vi "signal_analyze.vi"() -> ()   [LabVIEW 2021]
uses:
  <vilib>/express/express analysis/Spectral/Block/exnSpectralBlock spectral measurements power poly.vi
  <vilib>/express/express analysis/Spectral/Block/exnSpectralBlock spectral measurements power DDT.vi
  <vilib>/express/express analysis/Spectral/XNode/ExpressSpectralMeasurementsBlockNode.xnode
panel:
  in  "Stop":bool
  out "Waveform Graph":dynamicdata(graph)
  in  "Sine Frequency":dbl(knob) scale=0.0..500.0
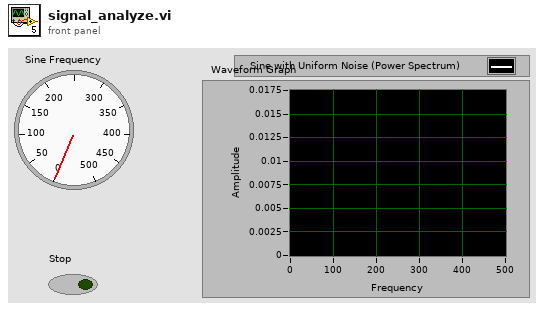
[diagram p1: front panel]
types:
  T1 = cluster{"averaging mode":u16, "weighting mode":u16, "number of averages":u32}
  T2 = cluster{"dB On (F)":bool, "unwrap phase (F)":bool, "convert to degree (F)":bool}
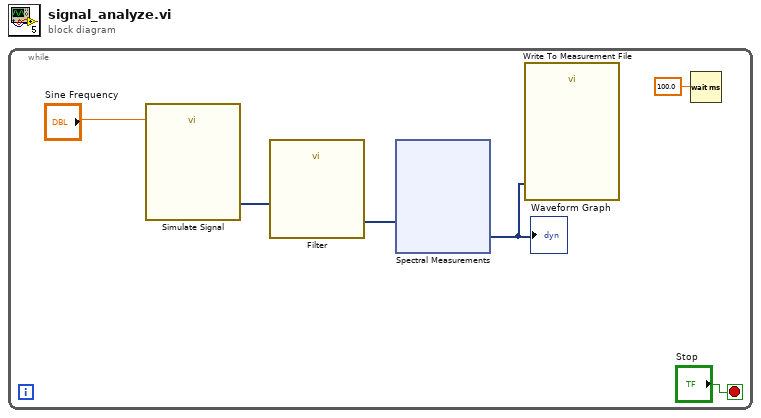
[diagram p0: block diagram]
diagram:
  n1 = while {
    stop <- "Stop" stop-if-true
    n2 = call "Simulate Signal"("Frequency"="Sine Frequency") -> ("Sine with Uniform Noise"=w5:dynamicdata)  [unwired: 13 in, 1 out]
    n3 = call "Filter"("Signal"=w5) -> ("Filtered Signal"=w4:dynamicdata)  [unwired: 9 in, 1 out]
    n4 = xnode "Spectral Measurements"("Signals"=w4) -> ("Power Spectrum"=w1:dynamicdata)  [unwired: 1 in, 1 out]
    "Waveform Graph" <- w1
    n5 = call "Write To Measurement File"("Signals"=w1) -> ()  [unwired: 16 in, 3 out]
    n6 = Wait (ms)(milliseconds to wait=100.0) -> ()  [unwired: 1 out]
  }
